vi "Initialize Tag from Waveform.vi"(8 "error in (no error)":errorcluster, 10 "Waveform in":waveform(dbl), 11 "Logger in.lvclass":refnum<class "Logger.lvclass">) -> (0 "error out":errorcluster, 2 "Waveform out":waveform(dbl), 3 "Logger out.lvclass":refnum<class "Logger.lvclass">)   [LabVIEW 2023, in "Logger.lvclass"]
uses:
  Logger.lvclass
  <vilib>/Skyline/Configuration/Workspace_class/NI SystemLink Workspace.lvclass/NI SystemLink Workspace.ctl
  Logger.lvclass/Logger.ctl
  <vilib>/Skyline/Tag/Shared/typedefs/TagProperty.ctl
  <vilib>/Skyline/Tag/Shared/typedefs/DataType.ctl
  <vilib>/Skyline/Tag/Wrapper/Wrapper_class/NI Skyline Tag.lvclass
  <vilib>/Skyline/Tag/Shared/typedefs/Retention Type.ctl
  <vilib>/Skyline/Configuration/Workspace_class/Read ID.vi
  <vilib>/Skyline/Utilities/Build Resource Name.vi
  <vilib>/Skyline/Tag/Shared/NI Skyline Tag.lvlib
  <vilib>/Skyline/Tag/Wrapper/Wrapper HTTP_class/NI Skyline Tag HTTP.lvclass
  <vilib>/Skyline/Utilities/NI Skyline Utilities.lvlib
  <vilib>/Skyline/Configuration/Workspace_class/NI SystemLink Workspace.lvclass
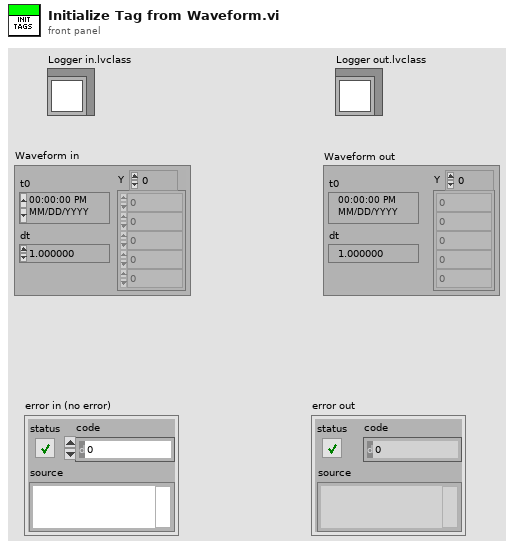
[diagram p1: front panel]
types:
  T1 = typedef "NI Skyline Tag.lvlib/Retention Type.ctl" = enum32{"None", "Duration", "Count", "Permanent"}
  T2 = cluster{"Tag Units":string, "Tag Path":string, "Tag Reference":refnum<class "NI Skyline Tag.lvclass">}
  T3 = typedef "NI Skyline Tag.lvlib/DataType.ctl" = enum32{"Double", "I32", "String", "Boolean", "U64", "Timestamp"}
  T4 = typedef "NI Skyline Tag.lvlib/TagProperty.ctl" = cluster{"key":string, "value":string}
  T5 = cluster{"Tag Units":string, "Tag Path":string, "Tag Reference":refnum<class "NI Skyline Tag.lvclass">}[]
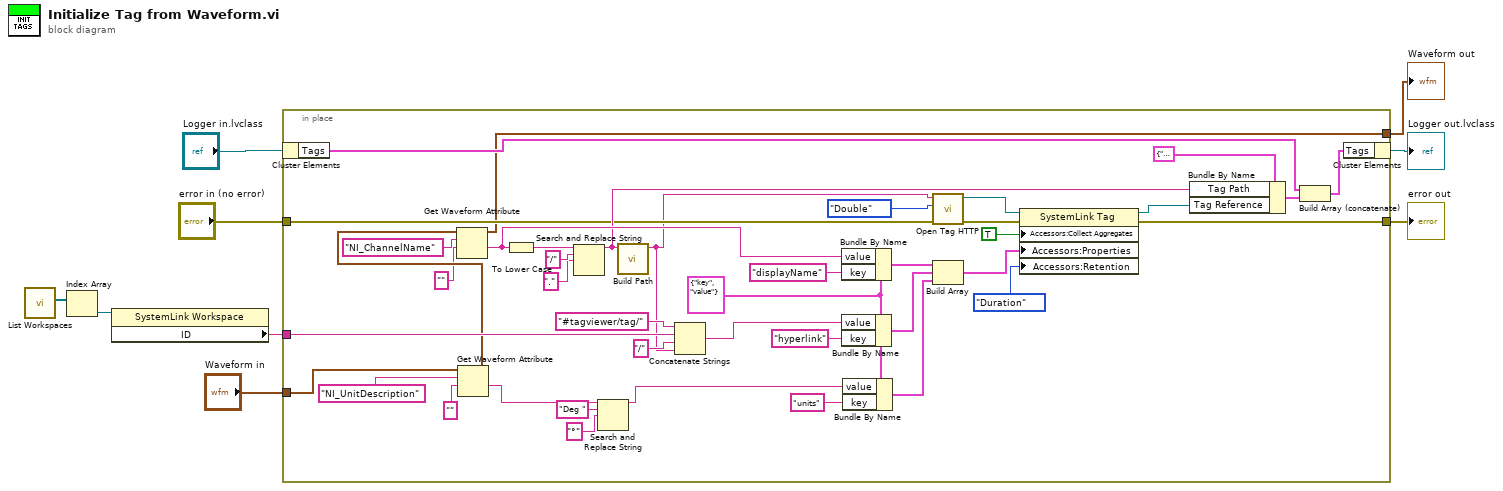
[diagram p0: block diagram]
diagram:
  n1 = call <vilib>:"List Workspaces.vi"() -> ("workspaces"=w3:refnum<class "NI SystemLink Workspace.lvclass">[])  [unwired: 9 in, 2 out]
  n2 = Index Array(array=w3) -> (element=w2:refnum<class "NI SystemLink Workspace.lvclass">)  [unwired: 1 in]
  n3 = property class="SystemLink Workspace"(reference=w2) -> ("ID"=w1:string)  [unwired: 1 in, 2 out]
  n4 = in-place {
    in-place-border: [w46] -> w9
    in-place-border: "error in (no error)" -> [w30]
    in-place-border: "Waveform in" -> [w19]
    in-place-border: [w20] -> w4
    in-place-border: w1 -> [w27]
    w21 = T4 {"key"="key", "value"="value"} ("Property")
    n5 = in-place-cluster #1("Logger in.lvclass") -> ("Tags"=w50:T5)
    n6 = Get Waveform Attribute(5:"", 6:"NI_UnitDescription" ("name"), 7:w19) -> (1:w13:string, 3:w18:waveform(dbl))  [unwired: 1 in, 2 out]
    n7 = Get Waveform Attribute(5:"", 6:"NI_ChannelName" ("name"), 7:w18) -> (1:w34:string, 3:w20:waveform(dbl))  [unwired: 1 in, 2 out]
    n8 = To Lower Case(string=w34) -> (all lower case string=w38:string)
    n9 = Search and Replace String(input string=w38, search string="/", replace string="." ("search string")) -> (result string=w33:string)  [unwired: 5 in, 3 out]
    n10 = Search and Replace String(input string=w13, search string="Deg ", replace string="°" ("replace string (\"\")")) -> (result string=w12:string)  [unwired: 5 in, 3 out]
    n11 = call <vilib>:"Build Path.vi"("tag name"=w33) -> ("path"=w25:string)  [unwired: 10 in]
    n12 = Concatenate Strings("#tagviewer/tag/", w27, "/" ("string"), w25) -> (w24:string)
    n13 = Bundle By Name(cluster=w21, "value"=w34, "key"="displayName") -> (w31:T4)
    n14 = Bundle By Name(cluster=w21, "value"=w24, "key"="hyperlink") -> (w23:T4)
    n15 = Bundle By Name(cluster=w21, "value"=w12, "key"="units") -> (w14:T4)
    n16 = call <vilib>:"Open Tag HTTP.vi"("error in (no error)"=w30, "Data Type"=DataType."Double", "path"=w25) -> ("error out"=w47:errorcluster, "tag"=w45:refnum<class "NI Skyline Tag.lvclass">)  [unwired: 7 in]
    n17 = Build Array(w31, w23, w14) -> (w43:T4[])
    n18 = property class="SystemLink Tag"(reference=w45, error in=w47, "Accessors:Collect Aggregates"=TRUE ("Collect Aggregates"), "Accessors:Properties"=w43, "Accessors:Retention"=Retention_Type."Duration" ("Retention")) -> (reference out=w44:refnum<class "NI Skyline Tag.lvclass">, error out=w46:errorcluster)
    n19 = Bundle By Name(cluster=T2 {"Tag Units"="", "Tag Path"="", "Tag Reference"=refnum} ("Tag"), "Tag Path"=w33, "Tag Reference"=w44) -> (w37:T2)
    n20 = Build Array (concatenate)(w50, w37) -> (w49:T5)
    n21 = in-place-cluster #1("Tags"=w49) -> (→"Logger out.lvclass":refnum<class "Logger.lvclass">)
  }
  "error out" <- w9
  "Waveform out" <- w4
